vi "draw missle.vi"(9 "new number of missles":i32, 10 "new missle position in":cluster{i32, i32, i32}[](array[cluster]), 11 "Board in":u32[][](array[numeric])) -> (2 "new missle position out":cluster{i32, i32, i32}[](array[cluster]), 3 "Board out":u32[][](array[numeric]))   [LabVIEW 2019]
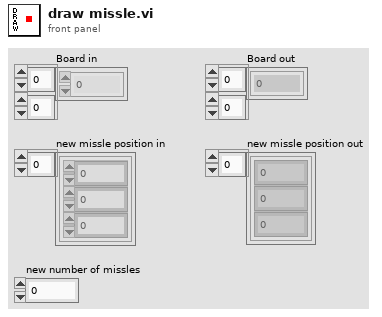
[diagram p1: front panel]
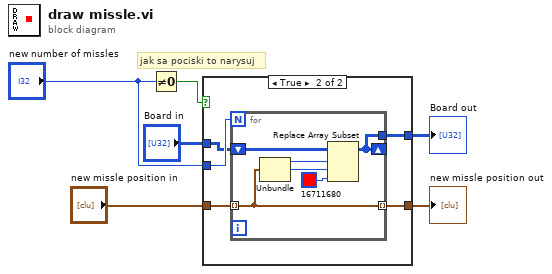
[diagram p0: block diagram]
diagram:
  # "jak sa pociski to narysuj"
  n1 = Not Equal To 0?(x="new number of missles") -> (x != 0?=w3:bool)
  n2 = case shown="True" w3 {
    tunnel: "new number of missles" -> [_ w13]
    tunnel: "Board in" -> [w8 w12]
    tunnel: "new missle position in" -> [w7 w11]
    tunnel: [w8 w10] -> w2
    tunnel: [w7 w9] -> w4
    frame False {
    }
    frame True {
      n3 = for {
        N: w13 -> [_]
        tunnel: w11 -> [w14] mode=indexing
        tunnel: [w15] -> w10
        shift-right: [w15] -> _
        shift-left: w12 -> [w19]
        tunnel: [w14] -> w9 mode=indexing
        n4 = Unbundle(w14) -> (w18:i32, w17:i32)  [unwired: 1 out]
        n5 = Replace Array Subset(array=w19, new element=u32 16711680, index (row)=w18, index (col)=w17) -> (w15:u32[][])
      }
    }
  }
  "new missle position out" <- w4
  "Board out" <- w2
